vi "setWaveforms.vi"(8 "error in (no error)":errorcluster, 11 "DAQmx in":refnum<class "DAQmx.lvclass">) -> (0 "error out":errorcluster, 3 "DAQmx out":refnum<class "DAQmx.lvclass">)   [LabVIEW 2019, in "DAQmx.lvclass"]
uses:
  DAQmx.lvclass
  typedefs/PrivateEvent--Waveforms--cluster.ctl
  DAQmx.lvclass/DAQmx.ctl
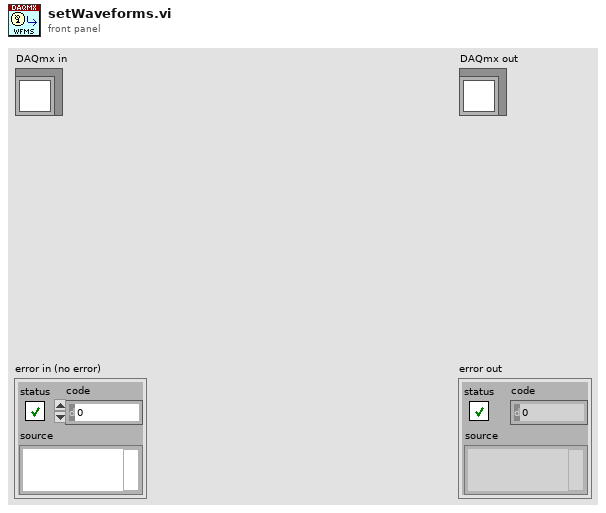
[diagram p1: front panel]
types:
  T1 = typedef "DAQmx.lvclass/PrivateEvent--Waveforms--cluster.ctl" = cluster{"AO":waveform(dbl)[], "AI":waveform(dbl)[], "REF_X":waveform(dbl)[], "REF_Y":waveform(dbl)[]}
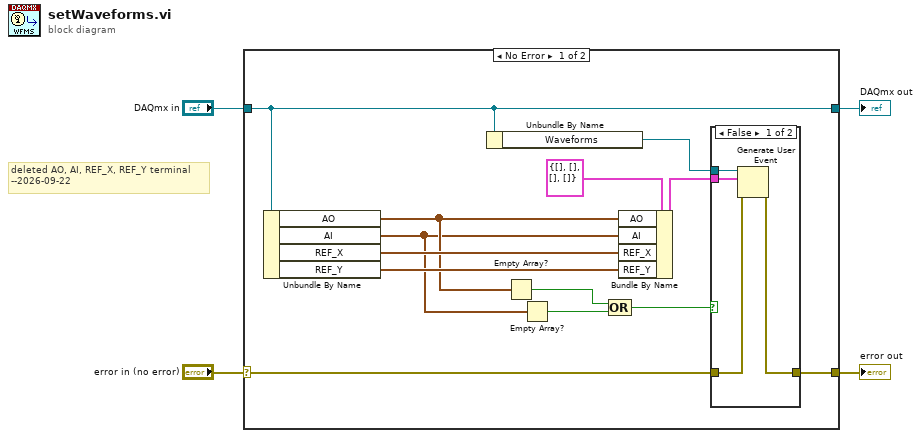
[diagram p0: block diagram]
diagram:
  # "deleted AO, AI, REF_X, REF_Y terminal\n--2026-09-22"
  n1 = case shown="No Error" "error in (no error)" {
    selector: "error in (no error)" -> [w17 w24]
    tunnel: [w16 w24] -> w3
    tunnel: [w9 w23] -> w1
    tunnel: "DAQmx in" -> [w9 w23]
    frame No Error {
      n2 = Unbundle By Name(w9) -> ("AO"=w6:waveform(dbl)[], "AI"=w5:waveform(dbl)[], "REF_X"=w7:waveform(dbl)[], "REF_Y"=w8:waveform(dbl)[])
      n3 = Unbundle By Name(w9) -> ("Waveforms"=w15:refnum<user-event>)
      n4 = Empty Array?(array=w6) -> (empty?=w12:bool)
      n5 = Empty Array?(array=w5) -> (empty?=w11:bool)
      n6 = Compound Arithmetic op=OR(w12, w11) -> (w10:bool)
      n7 = Bundle By Name(cluster=T1 {"AO"=[], "AI"=[], "REF_X"=[], "REF_Y"=[]} ("Waveforms"), "AO"=w6, "AI"=w5, "REF_X"=w7, "REF_Y"=w8) -> (w13:T1)
      n8 = case shown="False" w10 {
        tunnel: w17 -> [w21 w22]
        tunnel: [w20 w22] -> w16
        tunnel: w15 -> [w19 _]
        tunnel: w13 -> [w18 _]
        frame False {
          n9 = Generate User Event(user event=w19, event data cluster=w18, error in=w21) -> (error out=w20:errorcluster)  [unwired: 1 in, 1 out]
        }
        frame True {
        }
      }
    }
    frame Error {
    }
  }
  "error out" <- w3
  "DAQmx out" <- w1
